vi "runscenario export Report.vi"(8 "error in (no error)":errorcluster, 9 "POST (empty)":T1) -> (0 "error out":errorcluster, 1 "Export Filename":string, 2 "Export Content":string)   [LabVIEW 2011]
uses:
  ITK EXT/utils/keyedarr.llb/Keyed Array.ctl
  ITK EXT/utils/strutil.llb/Case Matching.ctl
  Summitek EXT/OpenG EXT/file/file.llb/Strip Path Extension - Path__ogtk.vi
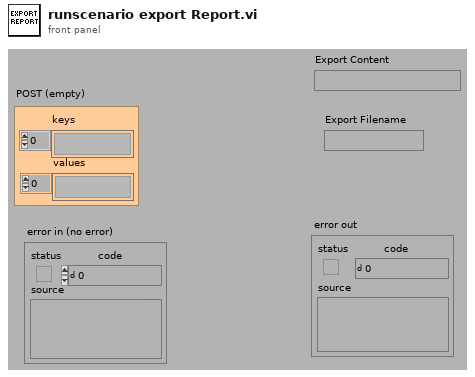
[diagram p1: front panel]
types:
  T1 = typedef "Keyed Array.ctl" = cluster{"keys":string[], "values":string[]}
  T2 = typedef "Case Matching.ctl" = enum16{"a != A", "a == A", "system"}
  T3 = enum16{"open", "replace", "create", "open or create", "replace or create", "replace or create with confirmation"}
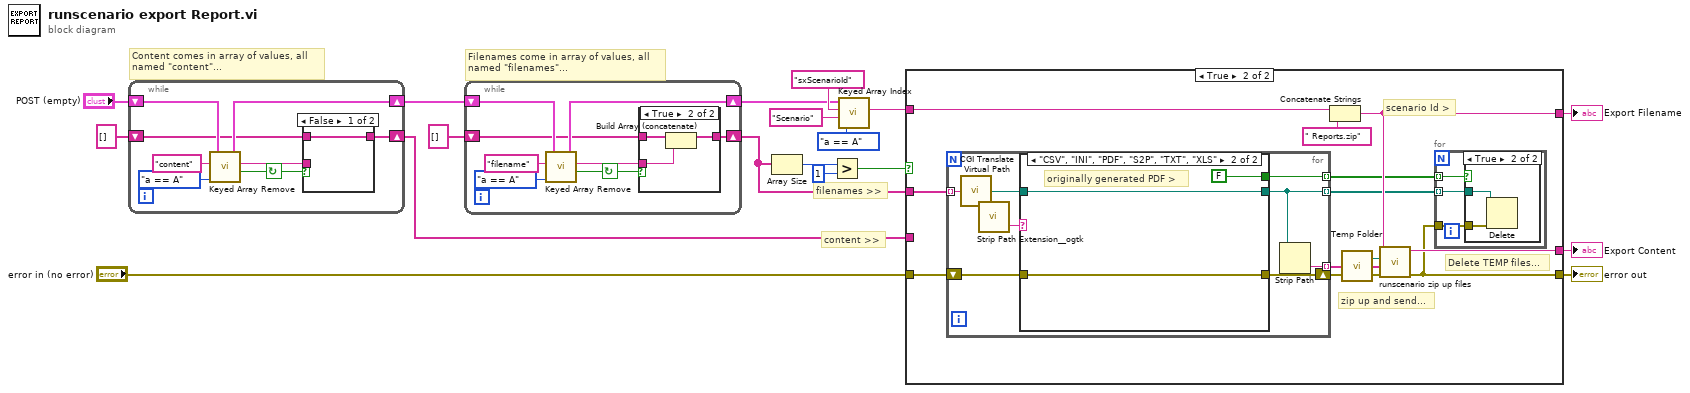
[diagram p0: block diagram]
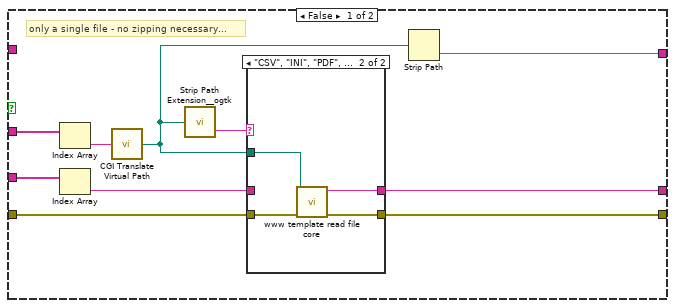
[diagram p3: hidden frame]
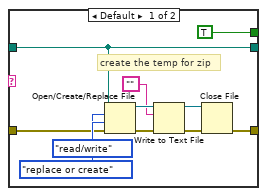
[diagram p6: hidden frame]
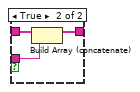
[diagram p7: hidden frame]
diagram:
  # "filenames >>"
  # "content >>"
  # "Filenames come in array of values, all\nnamed \"filenames\"..."
  # "Content comes in array of values, all\nnamed \"content\"..."
  n1 = while {
    shift-right: [w23] -> w5
    shift-left: "POST (empty)" -> [w24]
    shift-right: [w20] -> w14
    shift-left: string[] [] -> [w21]
    stop <- w22 continue-if-true
    n2 = call "Keyed Array Remove.vi"("case matching (sensitive)"=Case_Matching."a == A", "key"="content", "array in"=w24) -> ("valid key"=w22:bool, "value"=w19:string, "array out"=w23:T1)  [unwired: 2 out]
    n3 = case shown="False" w22 {
      tunnel: w21 -> [w27 w30]
      tunnel: [w27 w29] -> w20
      tunnel: w19 -> [_ w28]
      frame False {
      }
      frame True {
        n4 = Build Array (concatenate)(w30, w28) -> (w29:string[])
      }
    }
  }
  n5 = while {
    shift-right: [w35] -> w3
    shift-left: w5 -> [w36]
    shift-right: [w32] -> w1
    shift-left: string[] [] -> [w33]
    stop <- w34 continue-if-true
    n6 = call "Keyed Array Remove.vi"("case matching (sensitive)"=Case_Matching."a == A", "key"="filename", "array in"=w36) -> ("valid key"=w34:bool, "value"=w31:string, "array out"=w35:T1)  [unwired: 2 out]
    n7 = case shown="True" w34 {
      tunnel: w33 -> [w39 w42]
      tunnel: [w39 w41] -> w32
      tunnel: w31 -> [_ w40]
      frame False {
      }
      frame True {
        n8 = Build Array (concatenate)(w42, w40) -> (w41:string[])
      }
    }
  }
  n9 = Array Size(array=w1) -> (size(s)=w12:i32)
  n10 = Greater?(x=w12, y=1) -> (0:w15:bool)
  n11 = call "Keyed Array Index.vi"("case matching (sensitive)"=Case_Matching."a == A", "default value"="Scenario" ("key"), "key"="sxScenarioId", "array in"=w3) -> ("value"=w6:string)  [unwired: 3 out]
  n12 = case shown="True" w15 {
    tunnel: w14 -> [w52 _]
    tunnel: "error in (no error)" -> [w50 w69]
    tunnel: [w49 w61] -> w13
    tunnel: w6 -> [_ w60]
    tunnel: w1 -> [w51 w70]
    tunnel: [w47 w67] -> w11
    tunnel: [w45 w63] -> w10
    frame False {
      # "only a single file - no zipping necessary..."
      n13 = Index Array(array=w51) -> (element=w44:string)  [unwired: 1 in]
      n14 = Index Array(array=w52) -> (element=w48:string)  [unwired: 1 in]
      n15 = call "CGI Translate Virtual Path.vi"("virtual path"=w44) -> ("absolute path"=w43:path)  [unwired: 1 out]
      n16 = call-poly "Strip Path Extension__ogtk.vi"("path"=w43) -> ("extension"=w46:string)  [unwired: 1 out]
      n17 = case shown="\"CSV\", \"INI\", \"PDF\", \"S2P\", \"TXT\", \"XLS\"" w46 {
        tunnel: w50 -> [w53 w58]
        tunnel: [w53 w57] -> w49
        tunnel: w48 -> [w54 _]
        tunnel: [w54 w56] -> w47
        tunnel: w43 -> [_ w55]
        frame Default {
        }
        frame "CSV", "INI", "PDF", "S2P", "TXT", "XLS" {
          n18 = call "www template read file core.vi"("error in (no error)"=w58, "Path"=w55) -> ("error out"=w57:errorcluster, "File Content"=w56:string)  [unwired: 8 out]
        }
      }
      n19 = Strip Path(path=w43) -> (name=w45:string)  [unwired: 1 out]
    }
    frame True {
      # "scenario Id >"
      # "zip up and send..."
      # "Delete TEMP files..."
      n20 = for {
        tunnel: w70 -> [w77] mode=indexing
        shift-right: [w81] -> w68
        shift-left: w69 -> [w82]
        tunnel: [w79] -> w65 mode=indexing
        tunnel: [w80] -> w62 mode=indexing
        tunnel: [w78] -> w59 mode=indexing
        n21 = call "CGI Translate Virtual Path.vi"("virtual path"=w77) -> ("absolute path"=w76:path)  [unwired: 1 out]
        n22 = call-poly "Strip Path Extension__ogtk.vi"("path"=w76) -> ("extension"=w83:string)  [unwired: 1 out]
        n23 = case shown="\"CSV\", \"INI\", \"PDF\", \"S2P\", \"TXT\", \"XLS\"" w83 {
          tunnel: w82 -> [w90 w96]
          tunnel: [w89 w96] -> w81
          tunnel: w76 -> [w85 w97]
          tunnel: [w85 w97] -> w80
          tunnel: [TRUE FALSE] -> w78
          frame Default {
            # "create the temp for zip"
            n24 = Open/Create/Replace File(file path (use dialog)=w85, error in=w90, operation (0:open)=T3."replace or create", access (0:read/write)=enum16{"read/write", "read-only", "write-only"}."read/write") -> (refnum out=w87:refnum<file>, error out=w94:errorcluster)  [unwired: 3 out]
            n25 = Write to Text File(file (use dialog)=w87, text="", error in=w94) -> (refnum out=w88:refnum<file>, error out=w93:errorcluster)  [unwired: 2 out]
            n26 = Close File(refnum=w88, error in=w93) -> (error out=w89:errorcluster)  [unwired: 1 out]
          }
          frame "CSV", "INI", "PDF", "S2P", "TXT", "XLS" {
            # "originally generated PDF >"
          }
        }
        n27 = Strip Path(path=w80) -> (name=w79:string)  [unwired: 1 out]
      }
      n28 = Concatenate Strings(w60, " Reports.zip" ("format string")) -> (w63:string)
      n29 = call "Temp Folder.vi"() -> ("Temp Folder"=w66:path)  [unwired: 3 in]
      n30 = call "runscenario zip up files.vi"("error in (no error)"=w68, "Filenames to Zip (empty)"=w65, "Path to Files (empty)"=w66, "Zip filename (\"\")"=w63) -> ("error out"=w61:errorcluster, "Content"=w67:string)  [unwired: 6 out]
      n31 = for {
        tunnel: w62 -> [w72] mode=indexing
        tunnel: w61 -> [w73]
        tunnel: w59 -> [w71] mode=indexing
        n32 = case shown="True" w71 {
          tunnel: w72 -> [_ w75]
          tunnel: w73 -> [_ w74]
          frame False {
          }
          frame True {
            n33 = Delete(path (use dialog)=w75, error in=w74) -> ()  [unwired: 6 out]
          }
        }
      }
    }
  }
  "error out" <- w13
  "Export Content" <- w11
  "Export Filename" <- w10
